vi "Query S Parameters.vi"(8 "error in (no error)":errorcluster, 10 "Sparameters (string)":string[](array[string]), 11 "VNA-PNA in":refnum<class "VNA-PNA.lvclass">) -> (0 "error out":errorcluster, 2 "S parameters":T1[](array[typedef]), 3 "VNA-PNA out":refnum<class "VNA-PNA.lvclass">)   [LabVIEW 2020, in "VNA-PNA.lvclass"]
doc: "Queryes the S parameter choosen. It can give single parameter or full 2 to 4 port parameters.\nFor one port S Parameter array only have Sxx.\nFor N ports the S Parameter array hold S11,S12,...,S1N,S21,S22,...,SNN"
uses:
  VNA-PNA.lvclass
  C:/Sandbox/Git_Sandbox/WiSpry Test Framework source code (LV20)/WiSpry Test Framework/Instruments/Instrument.lvclass
  C:/Sandbox/Git_Sandbox/WiSpry Test Framework source code (LV20)/WiSpry Test Framework/Instruments/Vector Network Analyzer/Vector Network Analyzer.lvclass
  Controls/Sparameter cluster.ctl
  Instrument.lvclass/Instrument.ctl
  Vector Network Analyzer.lvclass/Vector Network Analyzer.ctl
  Instrument.lvclass
  Vector Network Analyzer.lvclass
panel:
  out "return count":u32
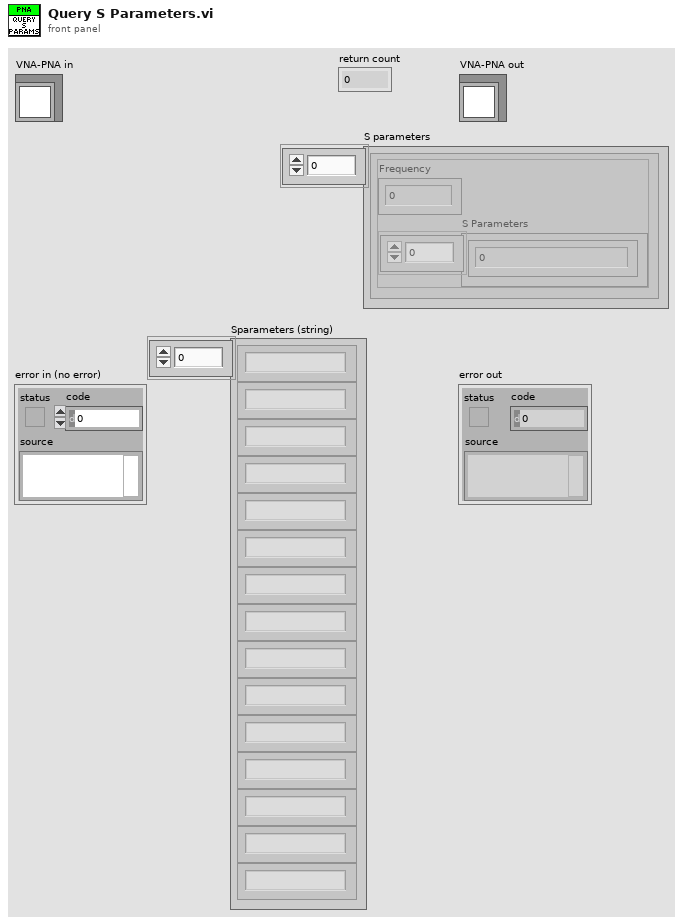
[diagram p1: front panel]
types:
  T1 = typedef "Vector Network Analyzer.lvclass/Sparameter cluster.ctl" = cluster{"Frequency":dbl, "S Parameters":cdb[]}
  T2 = enum16{"big-endian, network order", "native, host order", "little-endian"}
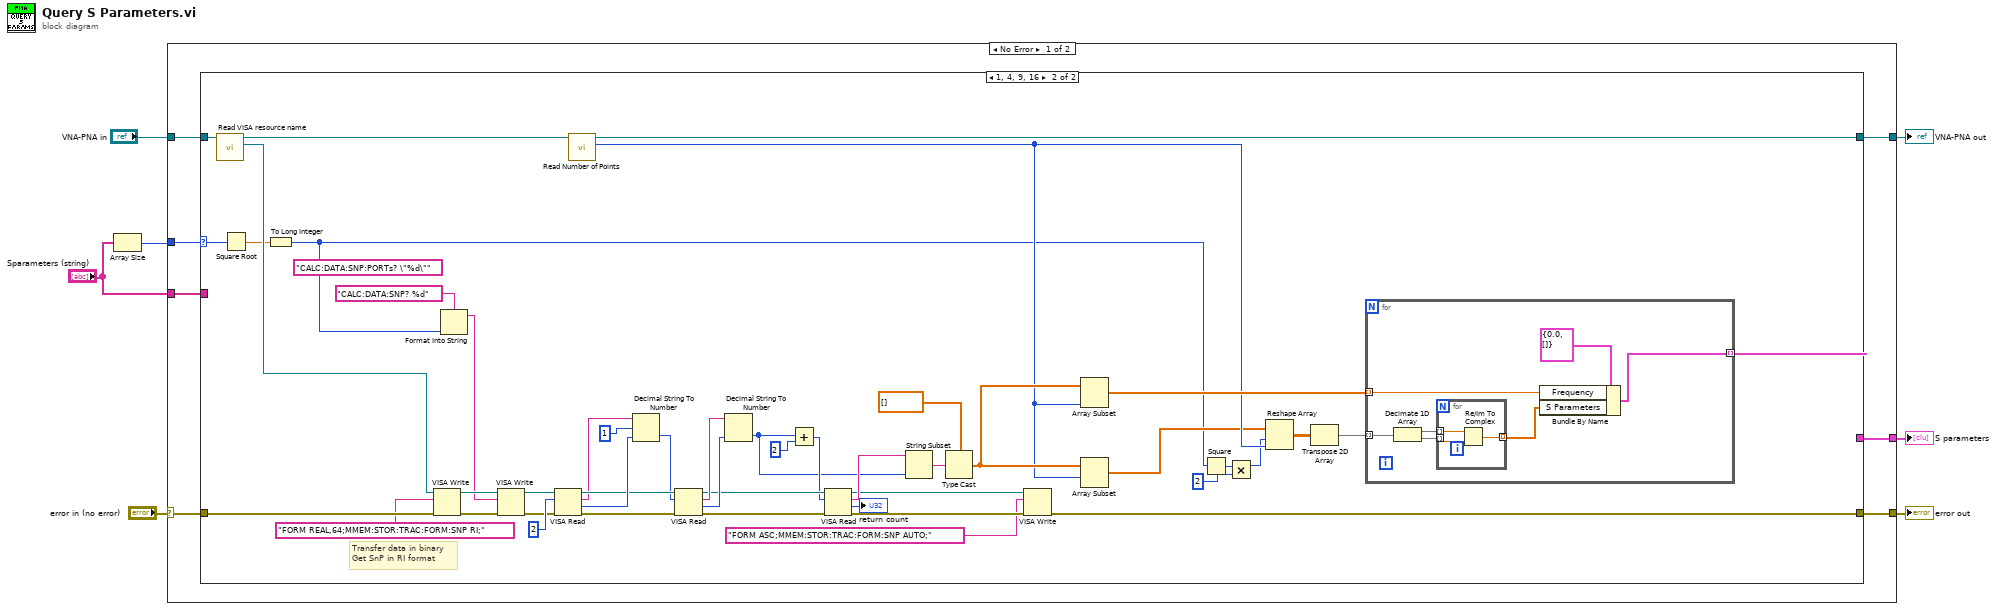
[diagram p0: block diagram]
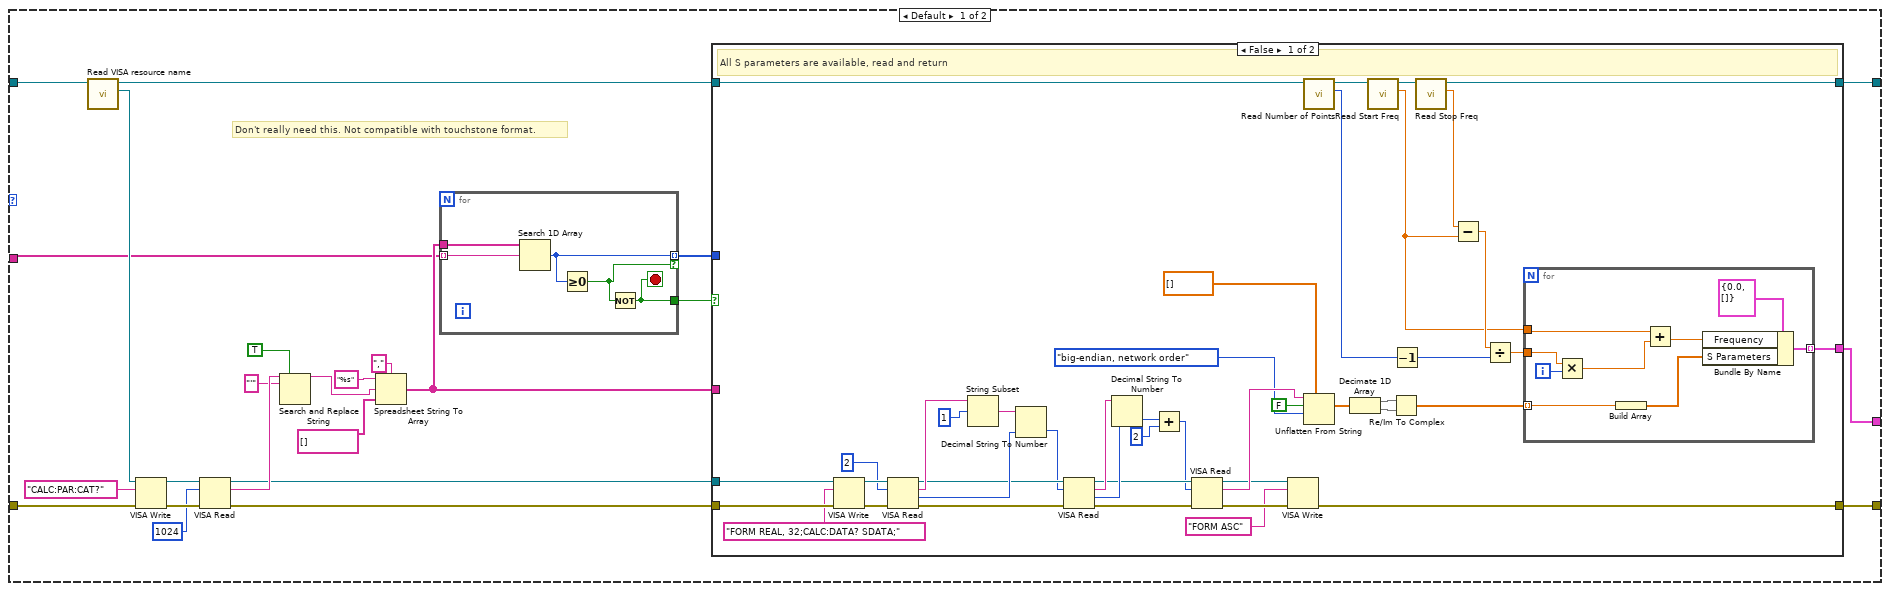
[diagram p2: hidden frame]
diagram:
  n1 = Array Size(array="Sparameters (string)") -> (size(s)=w1:i32)
  n2 = case shown="No Error" "error in (no error)" {
    selector: "error in (no error)" -> [w13 w156]
    tunnel: w1 -> [w9 _]
    tunnel: "VNA-PNA in" -> [w14 w155]
    tunnel: [w12 w155] -> w3
    tunnel: [w10 w156] -> w5
    tunnel: [w11 _] -> w4
    tunnel: "Sparameters (string)" -> [w8 _]
    frame No Error {
      n3 = case shown="1, 4, 9, 16" w9 {
        selector: w9 -> [_ w101]
        tunnel: w14 -> [w38 w144]
        tunnel: w13 -> [w37 w143]
        tunnel: [w21 w117] -> w12
        tunnel: [w20 w115] -> w11
        tunnel: [w16 w120] -> w10
        tunnel: w8 -> [w15 _]
        frame Default {
          # "Don't really need this. Not compatible with touchstone format."
          n4 = call "Read VISA resource name.vi"("Instrument in"=w38) -> ("VISA resource name"=w36:refnum<visa-resource-name>, "Instrument out"=w22:refnum<class "VNA-PNA.lvclass">)  [unwired: 9 in]
          n5 = VISA Write(VISA resource name=w36, write buffer="CALC:PAR:CAT?", error in (no error)=w37) -> (VISA resource name out=w33:refnum<visa-resource-name>, error out=w34:errorcluster)  [unwired: 1 out]
          n6 = VISA Read(VISA resource name=w33, byte count=u32 1024, error in (no error)=w34) -> (VISA resource name out=w23:refnum<visa-resource-name>, read buffer=w31:string, error out=w24:errorcluster)  [unwired: 1 out]
          n7 = Search and Replace String(replace all?=TRUE ("replace all? (F)"), input string=w31, search string="'") -> (result string=w26:string)  [unwired: 5 in, 3 out]
          n8 = Spreadsheet String To Array(delimiter (Tab)=",", format string="%s", spreadsheet string=w26, array type (2D Dbl)=string[] []) -> (array=w19:string[])
          n9 = for {
            tunnel: w15 -> [w96] mode=indexing
            tunnel: w19 -> [w97]
            tunnel: [w95] -> w18 mode=indexing if=w94
            tunnel: [w93] -> w17
            stop <- w93 stop-if-true
            n10 = Search 1D Array(1D array=w97, element=w96) -> (index of element=w95:i32)  [unwired: 1 in]
            n11 = Greater Or Equal To 0?(x=w95) -> (x >= 0?=w94:bool)
            n12 = Not(x=w94) -> (.not. x?=w93:bool)
          }
          n13 = case shown="False" w17 {
            tunnel: w24 -> [w81 w92]
            tunnel: w23 -> [w80 _]
            tunnel: w22 -> [w54 w91]
            tunnel: [w48 w91] -> w21
            tunnel: [w47 _] -> w20
            tunnel: w19 -> [_ _]
            tunnel: w18 -> [_ _]
            tunnel: [w40 w92] -> w16
            frame False {
              # "All S parameters are available, read and return"
              n14 = VISA Write(VISA resource name=w80, write buffer="FORM REAL, 32;CALC:DATA? SDATA;", error in (no error)=w81) -> (VISA resource name out=w77:refnum<visa-resource-name>, error out=w78:errorcluster)  [unwired: 1 out]
              n15 = VISA Read(VISA resource name=w77, byte count=u32 2, error in (no error)=w78) -> (VISA resource name out=w70:refnum<visa-resource-name>, read buffer=w73:string, return count=w72:u32, error out=w71:errorcluster)
              n16 = String Subset(string=w73, offset (0)=1) -> (substring=w74:string)  [unwired: 1 in]
              n17 = Decimal String To Number(string=w74, default (0L)=w72) -> (number=w69:u32)  [unwired: 1 in, 1 out]
              n18 = VISA Read(VISA resource name=w70, byte count=w69, error in (no error)=w71) -> (VISA resource name out=w64:refnum<visa-resource-name>, read buffer=w66:string, return count=w65:u32, error out=w62:errorcluster)
              n19 = Decimal String To Number(string=w66, default (0L)=w65) -> (number=w67:u32)  [unwired: 1 in, 1 out]
              n20 = Add(x=w67, y=u32 2) -> (x+y=w63:u32)
              n21 = VISA Read(VISA resource name=w64, byte count=w63, error in (no error)=w62) -> (VISA resource name out=w42:refnum<visa-resource-name>, read buffer=w61:string, error out=w43:errorcluster)  [unwired: 1 out]
              n22 = VISA Write(VISA resource name=w42, write buffer="FORM ASC", error in (no error)=w43) -> (error out=w40:errorcluster)  [unwired: 2 out]
              n23 = call "Read Number of Points.vi"("Vector Network Analyzer in"=w54) -> ("Number of Points"=w46:i32, "Vector Network Analyzer out"=w49:refnum<class "VNA-PNA.lvclass">)  [unwired: 9 in]
              n24 = Unflatten From String(type=dbl[] [], binary string=w61, data includes array or string size? (T)=FALSE, byte order (0:big-endian, network order)=T2."big-endian, network order") -> (value=w57:dbl[])  [unwired: 1 in, 2 out]
              n25 = Decimate 1D Array(w57) -> (w56:dbl[], w55:dbl[])
              n26 = call "Read Start Freq.vi"("Vector Network Analyzer in"=w49) -> ("Start Freq"=w44:dbl, "Vector Network Analyzer out"=w50:refnum<class "VNA-PNA.lvclass">)  [unwired: 9 in]
              n27 = Re/Im To Complex(1:w55, 2:w56) -> (0:w39:cdb[])
              n28 = Decrement(x=w46) -> (x-1=w45:i32)
              n29 = call "Read Stop Freq.vi"("Vector Network Analyzer in"=w50) -> ("Stop Freq"=w51:dbl, "Vector Network Analyzer out"=w48:refnum<class "VNA-PNA.lvclass">)  [unwired: 9 in]
              n30 = Subtract(x=w51, y=w44) -> (x-y=w52:dbl)
              n31 = Divide(x=w52, y=w45) -> (x/y=w53:dbl)
              n32 = for {
                tunnel: w44 -> [w87]
                tunnel: w53 -> [w89]
                tunnel: [w84] -> w47 mode=indexing
                tunnel: w39 -> [w83] mode=indexing
                i -> [w90]
                n33 = Multiply(x=w89, y=w90) -> (x*y=w88:dbl)
                n34 = Build Array(w83) -> (w82:cdb[])
                n35 = Add(x=w87, y=w88) -> (x+y=w85:dbl)
                n36 = Bundle By Name(cluster=T1 {"Frequency"=0.0, "S Parameters"=[]} ("S Parameters"), "Frequency"=w85, "S Parameters"=w82) -> (w84:T1)
              }
            }
            frame True {
              # "Add error handler"
              # "One of the parameters wanted is not available. Error"
            }
          }
        }
        frame 1, 4, 9, 16 {
          (unwired) "CALC:DATA:SNP:PORTs? \"%d\"" ("format string")
          # "Transfer data in binary\nGet SnP in RI format"
          n37 = call "Read VISA resource name.vi"("Instrument in"=w144) -> ("VISA resource name"=w106:refnum<visa-resource-name>, "Instrument out"=w118:refnum<class "VNA-PNA.lvclass">)  [unwired: 9 in]
          n38 = Square Root(x=w101) -> (sqrt(x)=w100:dbl)
          n39 = To Long Integer(number=w100) -> (32bit integer=w99:i32)
          n40 = VISA Write(VISA resource name=w106, write buffer="FORM REAL,64;MMEM:STOR:TRAC:FORM:SNP RI;", error in (no error)=w143) -> (VISA resource name out=w140:refnum<visa-resource-name>, error out=w141:errorcluster)  [unwired: 1 out]
          n41 = Format Into String(format string="CALC:DATA:SNP? %d", w99) -> (resulting string=w138:string)  [unwired: 2 in, 1 out]
          n42 = VISA Write(VISA resource name=w140, write buffer=w138, error in (no error)=w141) -> (VISA resource name out=w125:refnum<visa-resource-name>, error out=w126:errorcluster)  [unwired: 1 out]
          n43 = VISA Read(VISA resource name=w125, byte count=u32 2, error in (no error)=w126) -> (VISA resource name out=w134:refnum<visa-resource-name>, read buffer=w113:string, return count=w136:u32, error out=w135:errorcluster)
          n44 = call "Read Number of Points.vi"("Vector Network Analyzer in"=w118) -> ("Number of Points"=w108:i32, "Vector Network Analyzer out"=w117:refnum<class "VNA-PNA.lvclass">)  [unwired: 9 in]
          n45 = Decimal String To Number(string=w113, offset=1 ("offset (0)"), default (0L)=w136) -> (number=w133:u32)  [unwired: 1 out]
          n46 = VISA Read(VISA resource name=w134, byte count=w133, error in (no error)=w135) -> (VISA resource name out=w129:refnum<visa-resource-name>, read buffer=w131:string, return count=w130:u32, error out=w127:errorcluster)
          n47 = Decimal String To Number(string=w131, default (0L)=w130) -> (number=w119:u32)  [unwired: 1 in, 1 out]
          n48 = Add(x=w119, y=u32 2) -> (x+y=w128:u32)
          n49 = VISA Read(VISA resource name=w129, byte count=w128, error in (no error)=w127) -> (VISA resource name out=w122:refnum<visa-resource-name>, read buffer=w124:string, return count=→"return count":u32, error out=w123:errorcluster)
          n50 = String Subset(string=w124, length (rest)=w119) -> (substring=w111:string)  [unwired: 1 in]
          n51 = Type Cast(type=dbl[] [], x=w111) -> (*(type *) &x=w110:dbl[])
          n52 = VISA Write(VISA resource name=w122, write buffer="FORM ASC;MMEM:STOR:TRAC:FORM:SNP AUTO;", error in (no error)=w123) -> (error out=w120:errorcluster)  [unwired: 2 out]
          n53 = Array Subset(array=w110, length=w108) -> (w116:dbl[])  [unwired: 1 in]
          n54 = Array Subset(array=w110, index=w108) -> (w104:dbl[])  [unwired: 1 in]
          n55 = Square(x=w99) -> (x^2=w109:i32)
          n56 = Multiply(x=w109, y=2) -> (x*y=w103:i32)
          n57 = Reshape Array(w104, w103, w108) -> (w105:dbl[][])
          n58 = Transpose 2D Array(2D array=w105) -> (transposed array=w107:dbl[][])
          n59 = for {
            tunnel: w116 -> [w149] mode=indexing
            tunnel: w107 -> [w148] mode=indexing
            tunnel: [w150] -> w115 mode=indexing
            n60 = Decimate 1D Array(w148) -> (w147:dbl[], w146:dbl[])
            n61 = for {
              tunnel: w147 -> [w154] mode=indexing
              tunnel: w146 -> [w153] mode=indexing
              tunnel: [w152] -> w145 mode=indexing
              n62 = Re/Im To Complex(1:w153, 2:w154) -> (0:w152:cdb)
            }
            n63 = Bundle By Name(cluster=T1 {"Frequency"=0.0, "S Parameters"=[]} ("S Parameters"), "Frequency"=w149, "S Parameters"=w145) -> (w150:T1)
          }
        }
      }
    }
    frame Error {
    }
  }
  "error out" <- w5
  "VNA-PNA out" <- w3
  "S parameters" <- w4
